vi "Test Builder VIs.vi"() -> ()   [LabVIEW 2020]
uses:
  <vilib>/AppBuilder/AB_API_Simple/NI_App_Builder_API.lvlib
  <vilib>/AppBuilder/AB_API_Simple/Build (path).vi
panel:
  out "error out":errorcluster
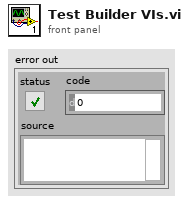
[diagram p1: front panel]
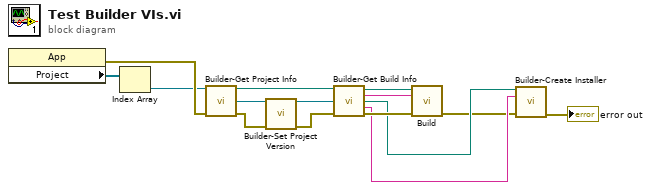
[diagram p0: block diagram]
diagram:
  n1 = property class="App"() -> (error out=w14:errorcluster, "Project"=w15:refnum<vi>[])  [unwired: 2 in, 1 out]
  n2 = Index Array(array=w15) -> (element=w12:refnum<vi>)  [unwired: 1 in]
  n3 = call "Builder-Get Project Info.vi"("Project ref"=w12, "error in (no error)"=w14) -> ("Project Path"=w10:path, "ProjectItem"=w9:refnum<vi>, "error out"=w13:errorcluster)  [unwired: 11 in]
  n4 = call "Builder-Set Project Version.vi"("ProjectItem in"=w9, "error in (no error)"=w13) -> ("ProjectItem out"=w8:refnum<vi>, "error out"=w11:errorcluster)  [unwired: 11 in, 1 out]
  n5 = call "Builder-Get Build Info.vi"("Project Path in"=w10, "Project Item"=w8, "error in (no error)"=w11) -> ("Project Path out"=w7:path, "Build Spec Name"=w6:string, "Exe Path"=w4:path, "Product Name"=w3:string, "error out"=w5:errorcluster)  [unwired: 8 in]
  n6 = call-poly <vilib>:"Build.vi"("error in (no error)"=w5, "Name of build specification (if empty: build all)"=w6, "Path to project"=w7) -> ("error out"=w1:errorcluster)  [unwired: 7 in, 1 out]
  n7 = call "Builder-Create Installer.vi"("Exe Path"=w4, "Product Name"=w3, "error in (no error)"=w1) -> ("error out"=→"error out":errorcluster)  [unwired: 11 in, 1 out]
